vi "GetSubjectUI.vi"(0 "Enable":bool=TRUE, 5 "error in (no error)":errorcluster) -> (14 "subjectSelected":string, 18 "OK":bool, 19 "error out":errorcluster)   [LabVIEW 2010]
doc: "Displays a standard dialog box that prompts users to enter information, such as a user name and password.\n--------------------\n\nThis Express VI is configured as follows:\n\nMessage to Display to the User:\nThe inputs are: \nCheckbox: Andy\nCheckbox: Apollo\nCheckbox: Ben\nCheckbox: Charles\nCheckbox: Claude\nCheckbox: Leo\nCheckbox: Woody"
panel:
  in  "Woody":bool
  in  "Leo":bool
  in  "Claude":bool
  in  "Charles":bool
  in  "Ben":bool
  in  "Apollo":bool
  in  "Andy":bool
  out "String":string
  in  "Cancel":bool
  in  "OK2":bool
  in  "OK1":bool
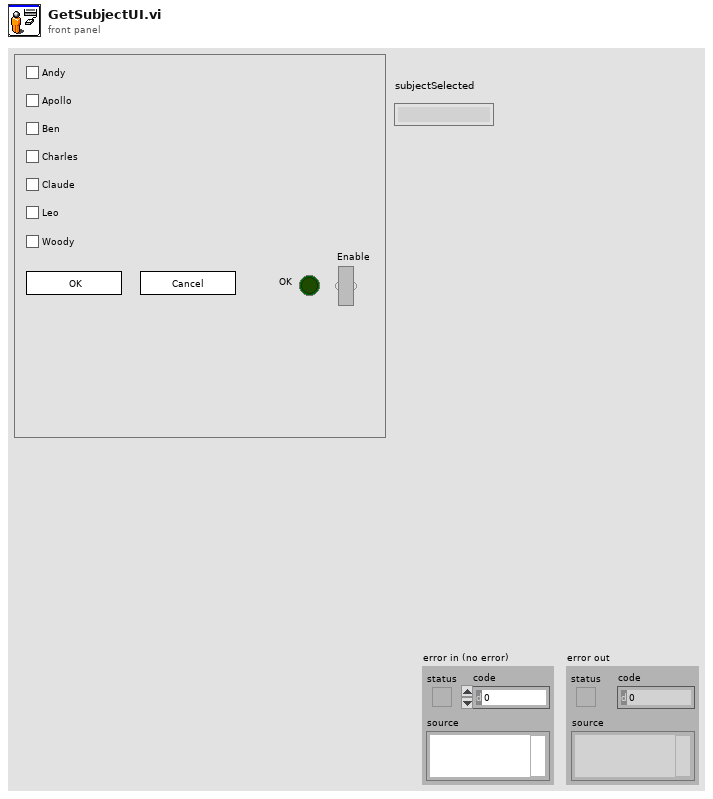
[diagram p1: front panel]
types:
  T1 = cluster{"Input Name":string, "Input Data Type":i32}[]
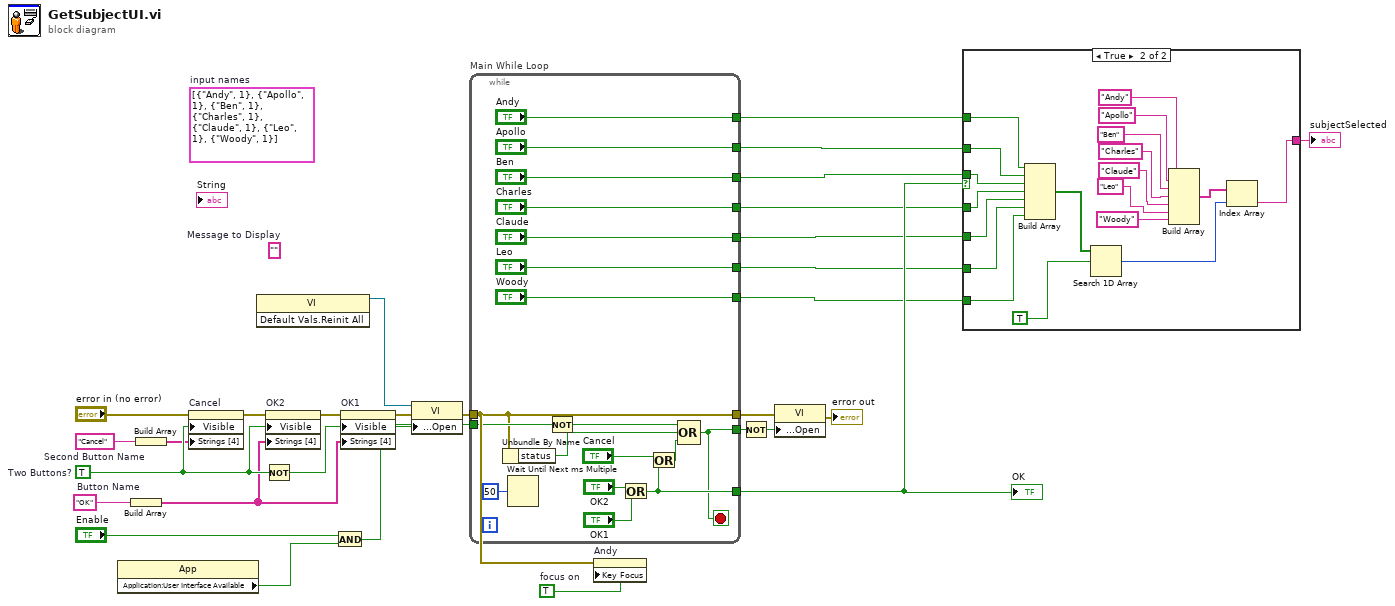
[diagram p0: block diagram]
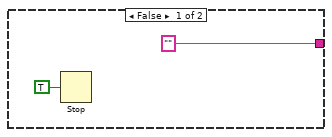
[diagram p2: hidden frame]
diagram:
  w10 = TRUE  # focus on
  (unwired) T1 [{"Input Name"="Andy", "Input Data Type"=1}, {"Input Name"="Apollo", "Input Data Type"=1}, {"Input Name"="Ben", "Input Data Type"=1}, {"Input Name"="Charles", "Input Data Type"=1}, {"Input Name"="Claude", "Input Data Type"=1}, {"Input Name"="Leo", "Input Data Type"=1}, {"Input Name"="Woody", "Input Data Type"=1}]  # input names
  w22 = "Cancel"  # Second Button Name
  w20 = "OK"  # Button Name
  (unwired) ""  # Message to Display
  w29 = TRUE  # Two Buttons?
  n1 = property class="App"() -> ("Application:User Interface Available"=w12:bool)  [unwired: 2 in, 2 out]
  n2 = Build Array(w20) -> (w21:string[])
  n3 = Build Array(w22) -> (w23:string[])
  n4 = property on="Cancel" class="Bool"(error in="error in (no error)", "Visible"=w29, "Strings [4]"=w23) -> (error out=w27:errorcluster)  [unwired: 1 in, 1 out]
  n5 = invoke class="VI" method="Default Vals.Reinit All"() -> (reference out=w11:refnum<vi>)  [unwired: 3 in, 2 out]
  n6 = Not(x=w29) -> (.not. x?=w28:bool)
  n7 = property on="OK2" class="Bool"(error in=w27, "Visible"=w29, "Strings [4]"=w21) -> (error out=w26:errorcluster)  [unwired: 1 in, 1 out]
  n8 = And(x="Enable", y=w12) -> (x .and. y?=w13:bool)
  n9 = property on="OK1" class="Bool"(error in=w26, "Visible"=w28, "Strings [4]"=w21) -> (error out=w19:errorcluster)  [unwired: 1 in, 1 out]
  n10 = property class="VI"(reference=w11, error in=w19, "Front Panel Window:Open"=w13) -> (error out=w18:errorcluster)  [unwired: 1 out]
  n11 = while "Main While Loop" {
    tunnel: [w44] -> w8
    tunnel: w13 -> [w42]
    tunnel: [w40] -> w24
    tunnel: w18 -> [w39]
    tunnel: [w39] -> w16
    tunnel: ["Andy"] -> w9
    tunnel: ["Apollo"] -> w7
    tunnel: ["Ben"] -> w6
    tunnel: ["Charles"] -> w5
    tunnel: ["Claude"] -> w4
    tunnel: ["Leo"] -> w3
    tunnel: ["Woody"] -> w2
    stop <- w40 stop-if-true
    n12 = Unbundle By Name(w39) -> ("status"=w37:bool)
    n13 = Wait Until Next ms Multiple(millisecond multiple=u32 50) -> ()  [unwired: 1 out]
    n14 = Not(x=w42) -> (.not. x?=w41:bool)
    n15 = Or(x="OK2", y="OK1") -> (x .or. y?=w44:bool)
    n16 = Or(x="Cancel", y=w44) -> (x .or. y?=w38:bool)
    n17 = Compound Arithmetic op=OR(w41, w37, w38) -> (w40:bool)
  }
  "OK" <- w8
  n18 = property on="Andy" class="Bool (strict)"(error in=w18, "Key Focus"=w10) -> ()  [unwired: 1 in, 2 out]
  n19 = Not(x=w24) -> (.not. x?=w25:bool)
  n20 = property class="VI"(error in=w16, "Front Panel Window:Open"=w25) -> (error out=→"error out":errorcluster)  [unwired: 1 in, 1 out]
  n21 = case shown="True" w8 {
    tunnel: ["" w60] -> w1
    tunnel: w9 -> [_ w57]
    tunnel: w7 -> [_ w56]
    tunnel: w6 -> [_ w55]
    tunnel: w5 -> [_ w54]
    tunnel: w4 -> [_ w53]
    tunnel: w3 -> [_ w52]
    tunnel: w2 -> [_ w51]
    frame False {
      n22 = Stop(stop? (T)=TRUE) -> ()
    }
    frame True {
      n23 = Build Array(w57, w56, w55, w54, w53, w52, w51) -> (w59:bool[])
      n24 = Search 1D Array(1D array=w59, element=TRUE) -> (index of element=w58:i32)  [unwired: 1 in]
      n25 = Build Array("Andy", "Apollo", "Ben", "Charles", "Claude", "Leo", "Woody") -> (w68:string[])
      n26 = Index Array(array=w68, index=w58) -> (element=w60:string)
    }
  }
  "subjectSelected" <- w1
